vi "send mail.vi"(6 "Mail Server":string="mailout.natinst.com", 7 "TO: [Mail_Reciepient]":string[](array[string]), 8 "error in":errorcluster, 9 "Subject  For Email":string="[No Subject]", 10 "From [Sender Email]":string, 11 "LogFile path":path) -> (0 "error out":errorcluster, 4 "invalid recipients":string[](array[string]), 5 "Body Of E-mail":string)   [LabVIEW 2015]
uses:
  <vilib>/Utility/SMTP/NI_SMTPEmail.lvlib
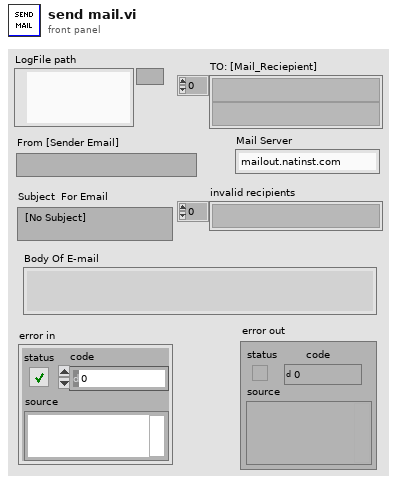
[diagram p1: front panel]
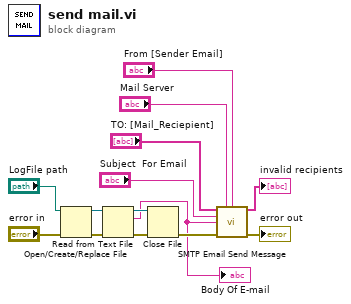
[diagram p0: block diagram]
diagram:
  n1 = Open/Create/Replace File(file path (use dialog)="LogFile path", error in="error in") -> (refnum out=w12:refnum<file>, error out=w10:errorcluster)  [unwired: 4 in, 1 out]
  n2 = Read from Text File(file (use dialog)=w12, error in=w10) -> (refnum out=w11:refnum<file>, text=w7:string, error out=w9:errorcluster)  [unwired: 2 in, 1 out]
  "Body Of E-mail" <- w7
  n3 = Close File(refnum=w11, error in=w9) -> (error out=w8:errorcluster)  [unwired: 1 out]
  n4 = call <vilib>:"SMTP Email Send Message.vi"("recipients"="TO: [Mail_Reciepient]", "mail server"="Mail Server", "return address"="From [Sender Email]", "subject ([No Subject])"="Subject  For Email", "message"=w7, "error in (no error)"=w8) -> ("invalid recipients"=→"invalid recipients":string[], "error out"=→"error out":errorcluster)  [unwired: 8 out]
